vi "Enable Current Sharing.vi"(8 "error in (no error)":errorcluster, 11 "69X_79X in":refnum<class "6972A.lvclass">) -> (0 "error out":errorcluster, 3 "69X_79X out":refnum<class "6972A.lvclass">)   [LabVIEW 2019, in "6972A.lvlib" / "6972A.lvclass"]
uses:
  Library/6972A.lvclass
  C:/Users/Public/Documents/Development/builds/Instruments/PowerSupply.lvlibp/Library/PowerSupply.lvclass
  Library/6972A.lvclass/6972A.ctl
  Accessors/Read Local Resource.vi
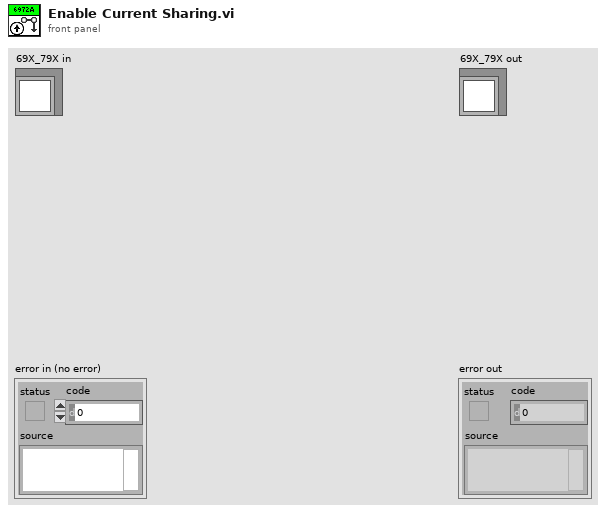
[diagram p1: front panel]
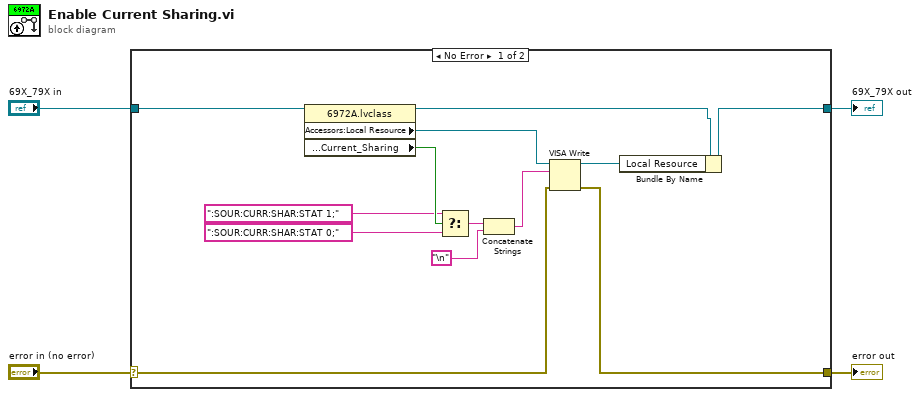
[diagram p0: block diagram]
diagram:
  n1 = case shown="No Error" "error in (no error)" {
    selector: "error in (no error)" -> [w15 w19]
    tunnel: [w14 w19] -> w3
    tunnel: [w17 w18] -> w1
    tunnel: "69X_79X in" -> [w13 w18]
    frame No Error {
      n2 = property class="6972A.lvclass"(reference=w13) -> (reference out=w12:refnum<class "6972A.lvclass">, "Accessors:Local Resource"=w11:refnum<visa-resource-name>, "Accessors:Setting:Current_Sharing"=w9:bool)  [unwired: 1 in, 1 out]
      n3 = Select(t=":SOUR:CURR:SHAR:STAT 1;" ("format string"), s=w9, f=":SOUR:CURR:SHAR:STAT 0;" ("format string")) -> (s? t:f=w10:string)
      n4 = Concatenate Strings(w10, "\n") -> (w6:string)
      n5 = VISA Write(VISA resource name=w11, write buffer=w6, error in (no error)=w15) -> (VISA resource name out=w16:refnum<visa-resource-name>, error out=w14:errorcluster)  [unwired: 1 out]
      n6 = Bundle By Name(cluster=w12, "Local Resource"=w16) -> (w17:refnum<class "6972A.lvclass">)
    }
    frame Error {
    }
  }
  "error out" <- w3
  "69X_79X out" <- w1
